vi "initialisationHWError.vi"(8 "error in (no error)":errorcluster, 11 "AtomChipHWC in":refnum<class "AtomChipHWC.lvclass">) -> (0 "error out":errorcluster, 3 "AtomChipHWC out":refnum<class "AtomChipHWC.lvclass">)   [LabVIEW 2011, in "Hardware.lvlib" / "HWControllers.lvlib" / "AtomChipHWC.lvclass"]
uses:
  AtomChipHWC.lvclass
  AtomChipHWC.lvclass/AtomChipHWC.ctl
  Channels/Digital/DigitalOutput.lvclass
  Channels/VoltOutput/AnalogOutput.lvclass
  Channels/DDSOutput/Generic/DDSOutput.lvclass
  Network Controllers/NetworkCamera/NetworkCamera.lvclass
  HWController.lvclass
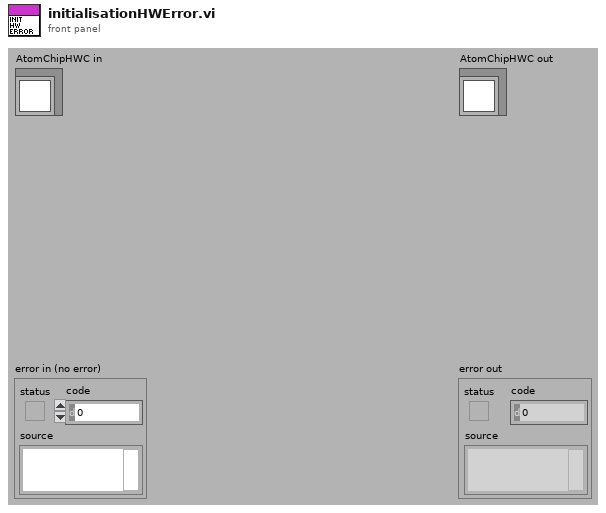
[diagram p1: front panel]
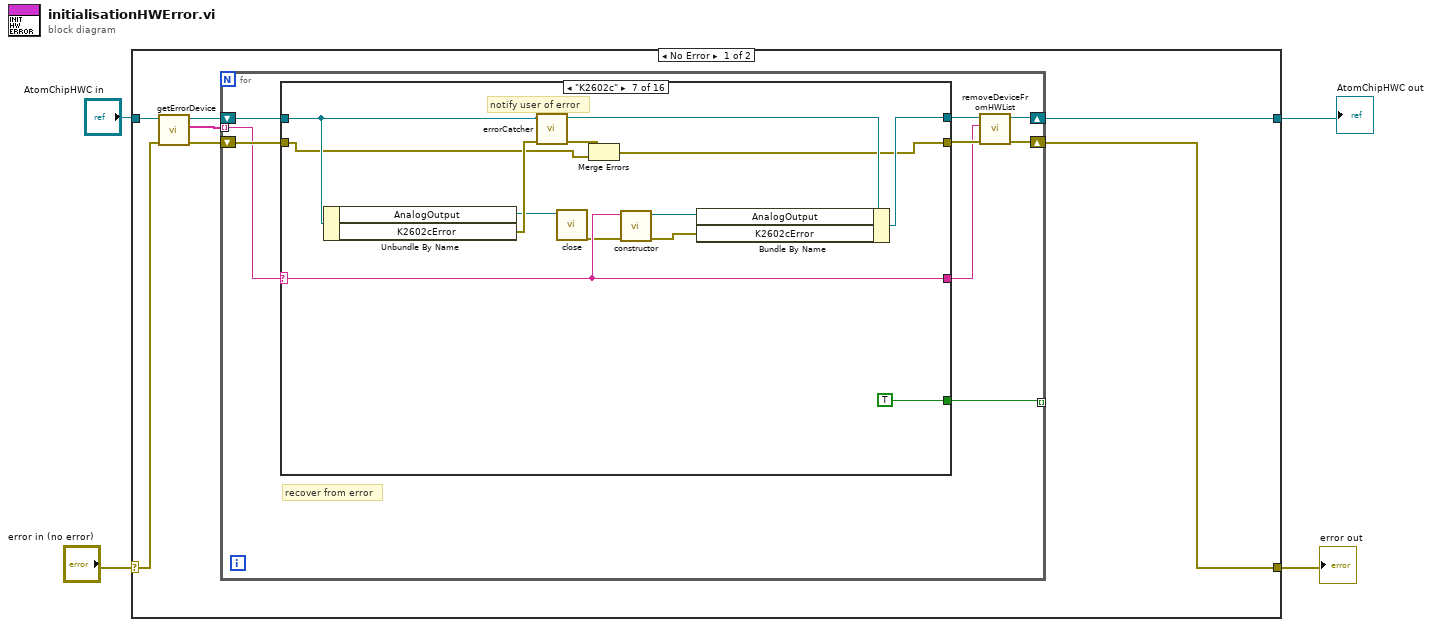
[diagram p0: block diagram]
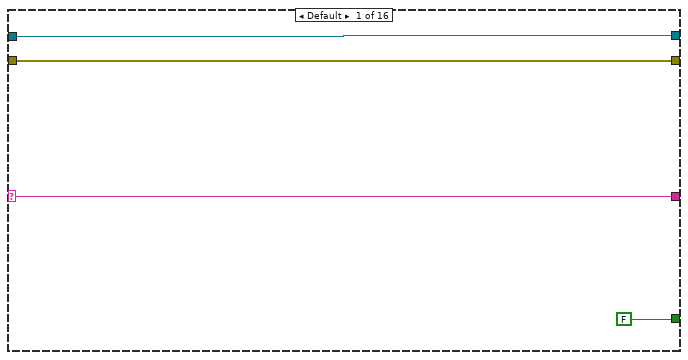
[diagram p2: hidden frame]
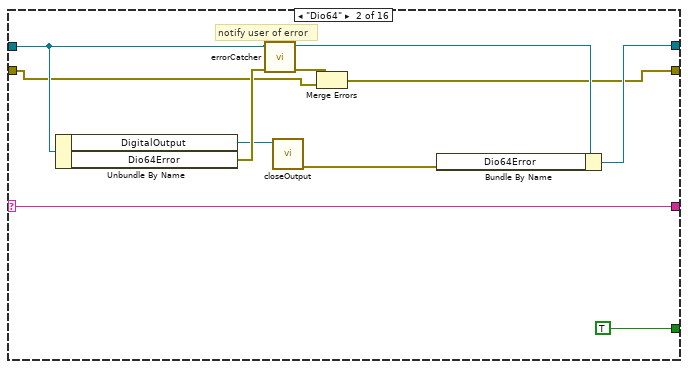
[diagram p3: hidden frame]
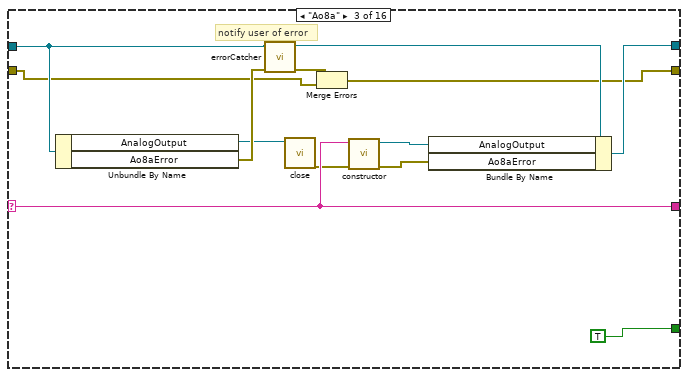
[diagram p4: hidden frame]
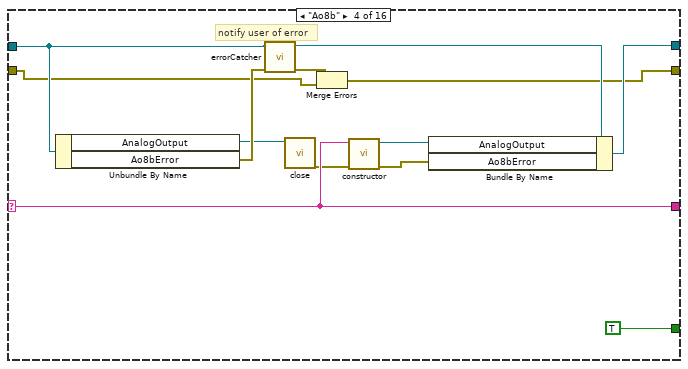
[diagram p5: hidden frame]
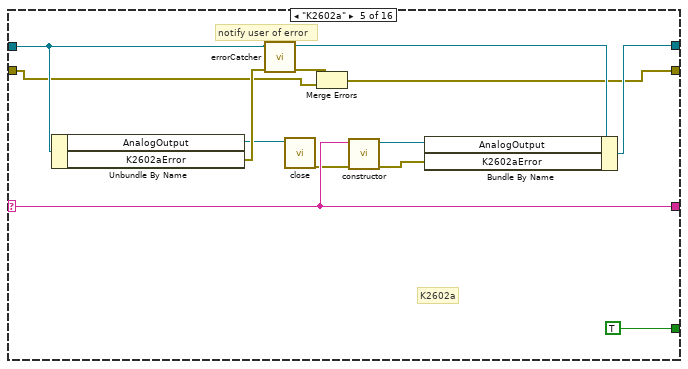
[diagram p6: hidden frame]
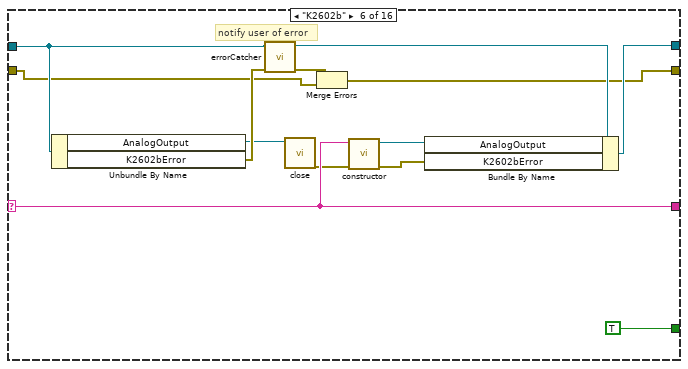
[diagram p7: hidden frame]
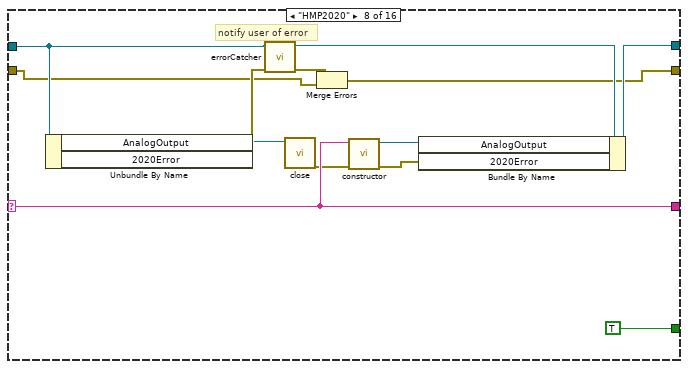
[diagram p8: hidden frame]
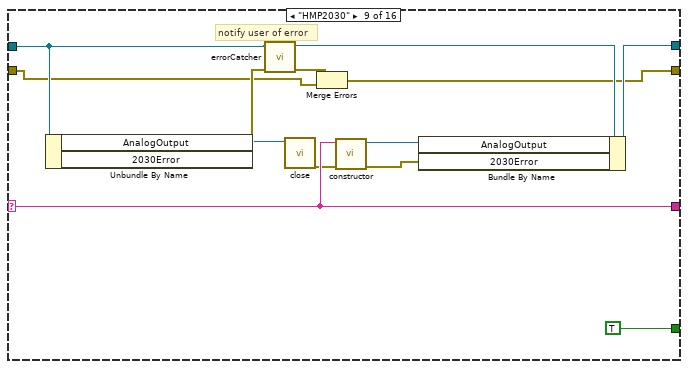
[diagram p9: hidden frame]
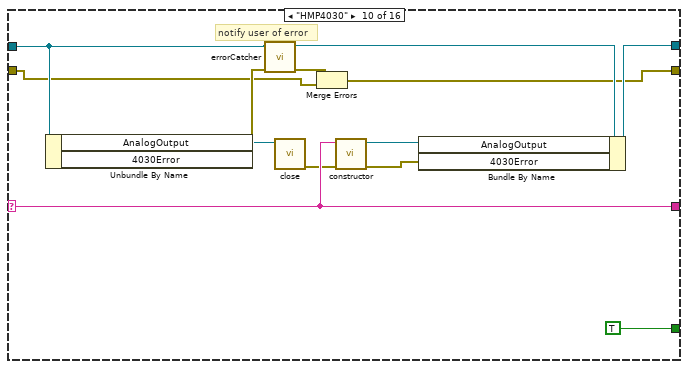
[diagram p10: hidden frame]
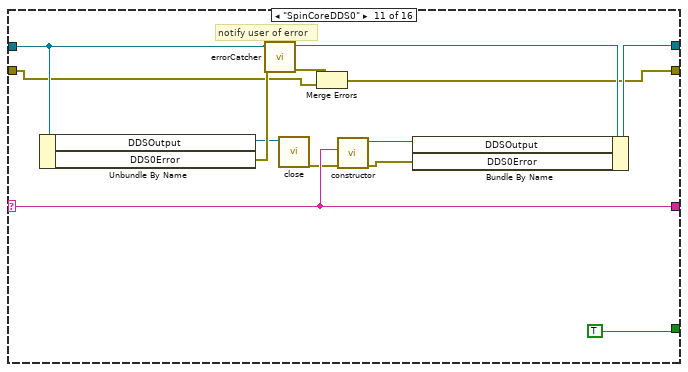
[diagram p11: hidden frame]
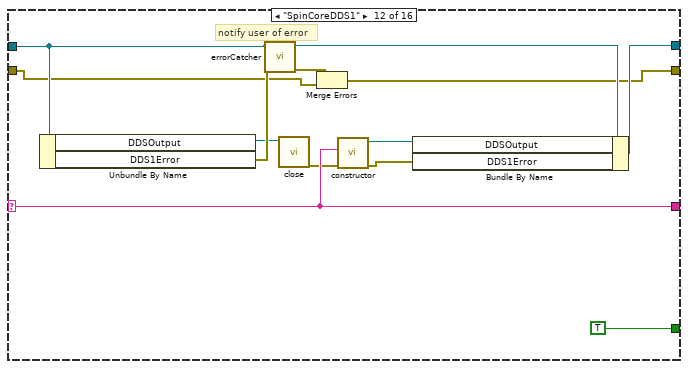
[diagram p12: hidden frame]
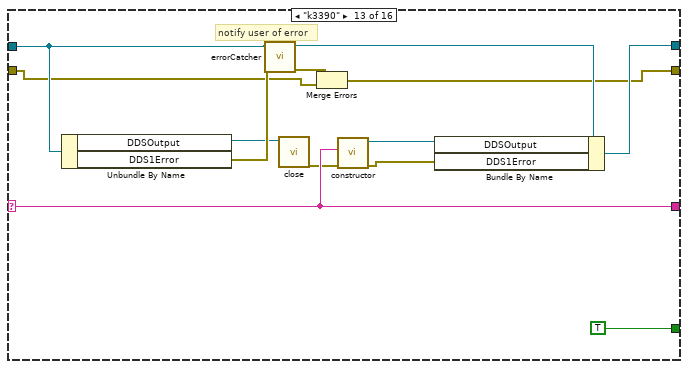
[diagram p13: hidden frame]
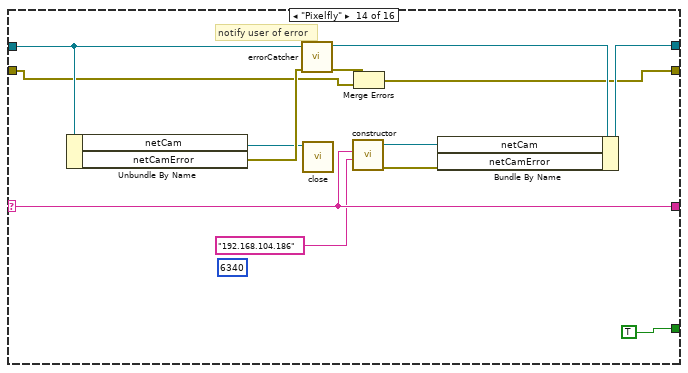
[diagram p14: hidden frame]
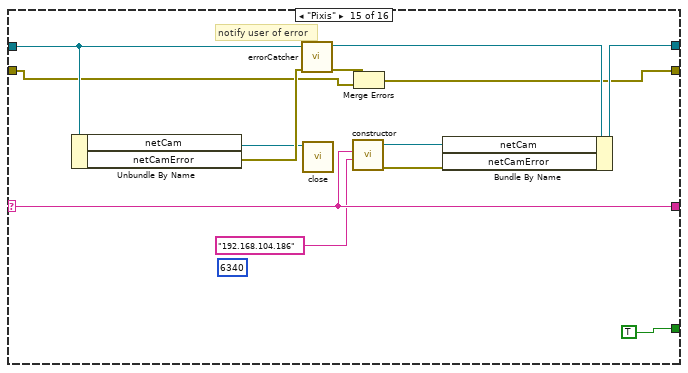
[diagram p15: hidden frame]
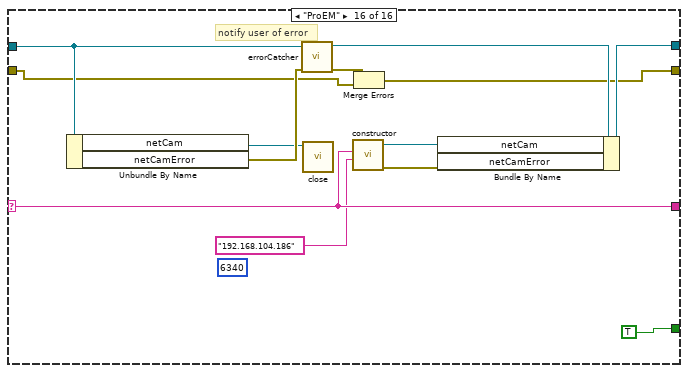
[diagram p16: hidden frame]
diagram:
  n1 = case shown="No Error" "error in (no error)" {
    selector: "error in (no error)" -> [w10 w218]
    tunnel: "AtomChipHWC in" -> [w11 w219]
    tunnel: [w6 w219] -> w2
    tunnel: [w5 w218] -> w1
    frame No Error {
      n2 = call "getErrorDevice.vi"("error in (no error)"=w10, "AtomChipHWC in"=w11) -> ("error out"=w7:errorcluster, "Devices"=w8:string[], "AtomChipHWC out"=w9:refnum<class "AtomChipHWC.lvclass">)  [unwired: 7 in]
      n3 = for {
        tunnel: w8 -> [w18] mode=indexing
        shift-right: [w14] -> w6
        shift-left: w9 -> [w20]
        shift-right: [w13] -> w5
        shift-left: w7 -> [w19]
        tunnel: [w12] -> _ mode=indexing
        # "recover from error"
        n4 = case shown="\"K2602c\"" w18 {
          selector: w18 -> [w22 w28 w40 w53 w66 w79 w92 w105 w118 w131 w142 w155 w168 w182 w195 w208]
          tunnel: w20 -> [w24 w35 w48 w61 w74 w87 w100 w113 w126 w139 w152 w165 w178 w191 w204 w217]
          tunnel: [w24 w30 w43 w56 w69 w82 w95 w108 w121 w134 w147 w160 w173 w186 w199 w212] -> w17
          tunnel: [w23 w29 w42 w55 w68 w81 w94 w107 w120 w133 w146 w159 w172 w185 w198 w211] -> w16
          tunnel: w19 -> [w23 w31 w44 w57 w70 w83 w96 w109 w122 w135 w148 w161 w174 w187 w200 w213]
          tunnel: [w22 w28 w40 w53 w66 w79 w92 w105 w118 w131 w142 w155 w168 w182 w195 w208] -> w15
          tunnel: [FALSE TRUE TRUE TRUE TRUE TRUE TRUE TRUE TRUE TRUE TRUE TRUE TRUE TRUE TRUE TRUE] -> w12
          frame Default {
          }
          frame "Dio64" {
            # "notify user of error"
            n5 = Unbundle By Name(w35) -> ("DigitalOutput"=w26:refnum<class "DigitalOutput.lvclass">, "Dio64Error"=w33:errorcluster)
            n6 = call-dynamic "errorCatcher.vi"("error in (no error)"=w33, "HWController in"=w35) -> ("error out"=w32:errorcluster, "HWController out"=w34:refnum<class "AtomChipHWC.lvclass">)  [unwired: 8 in]
            n7 = call-dynamic "closeOutput.vi"("DigitalOutput in"=w26) -> ("error out"=w27:errorcluster)  [unwired: 10 in]
            n8 = Merge Errors(w32, w31) -> (w29:errorcluster)
            n9 = Bundle By Name(cluster=w34, "Dio64Error"=w27) -> (w30:refnum<class "AtomChipHWC.lvclass">)
          }
          frame "Ao8a" {
            # "notify user of error"
            n10 = Unbundle By Name(w48) -> ("AnalogOutput"=w41:refnum<class "AnalogOutput.lvclass">, "Ao8aError"=w46:errorcluster)
            n11 = call-dynamic "errorCatcher.vi"("error in (no error)"=w46, "HWController in"=w48) -> ("error out"=w45:errorcluster, "HWController out"=w47:refnum<class "AtomChipHWC.lvclass">)  [unwired: 8 in]
            n12 = call-dynamic "close.vi"("AnalogOutput in"=w41) -> ("error out"=w39:errorcluster)  [unwired: 10 in]
            n13 = Merge Errors(w45, w44) -> (w42:errorcluster)
            n14 = call "constructor.vi"("error in (no error)"=w39, "deviceName"=w40) -> ("error out"=w37:errorcluster, "AnalogOutput out"=w38:refnum<class "AnalogOutput.lvclass">)  [unwired: 8 in]
            n15 = Bundle By Name(cluster=w47, "AnalogOutput"=w38, "Ao8aError"=w37) -> (w43:refnum<class "AtomChipHWC.lvclass">)
          }
          frame "Ao8b" {
            # "notify user of error"
            n16 = Unbundle By Name(w61) -> ("AnalogOutput"=w54:refnum<class "AnalogOutput.lvclass">, "Ao8bError"=w59:errorcluster)
            n17 = call-dynamic "errorCatcher.vi"("error in (no error)"=w59, "HWController in"=w61) -> ("error out"=w58:errorcluster, "HWController out"=w60:refnum<class "AtomChipHWC.lvclass">)  [unwired: 8 in]
            n18 = call-dynamic "close.vi"("AnalogOutput in"=w54) -> ("error out"=w52:errorcluster)  [unwired: 10 in]
            n19 = Merge Errors(w58, w57) -> (w55:errorcluster)
            n20 = call "constructor.vi"("error in (no error)"=w52, "deviceName"=w53) -> ("error out"=w50:errorcluster, "AnalogOutput out"=w51:refnum<class "AnalogOutput.lvclass">)  [unwired: 8 in]
            n21 = Bundle By Name(cluster=w60, "AnalogOutput"=w51, "Ao8bError"=w50) -> (w56:refnum<class "AtomChipHWC.lvclass">)
          }
          frame "K2602a" {
            # "K2602a"
            # "notify user of error"
            n22 = Unbundle By Name(w74) -> ("AnalogOutput"=w67:refnum<class "AnalogOutput.lvclass">, "K2602aError"=w72:errorcluster)
            n23 = call-dynamic "errorCatcher.vi"("error in (no error)"=w72, "HWController in"=w74) -> ("error out"=w71:errorcluster, "HWController out"=w73:refnum<class "AtomChipHWC.lvclass">)  [unwired: 8 in]
            n24 = call-dynamic "close.vi"("AnalogOutput in"=w67) -> ("error out"=w65:errorcluster)  [unwired: 10 in]
            n25 = Merge Errors(w71, w70) -> (w68:errorcluster)
            n26 = call "constructor.vi"("error in (no error)"=w65, "deviceName"=w66) -> ("error out"=w63:errorcluster, "AnalogOutput out"=w64:refnum<class "AnalogOutput.lvclass">)  [unwired: 8 in]
            n27 = Bundle By Name(cluster=w73, "AnalogOutput"=w64, "K2602aError"=w63) -> (w69:refnum<class "AtomChipHWC.lvclass">)
          }
          frame "K2602b" {
            # "notify user of error"
            n28 = Unbundle By Name(w87) -> ("AnalogOutput"=w80:refnum<class "AnalogOutput.lvclass">, "K2602bError"=w85:errorcluster)
            n29 = call-dynamic "errorCatcher.vi"("error in (no error)"=w85, "HWController in"=w87) -> ("error out"=w84:errorcluster, "HWController out"=w86:refnum<class "AtomChipHWC.lvclass">)  [unwired: 8 in]
            n30 = call-dynamic "close.vi"("AnalogOutput in"=w80) -> ("error out"=w78:errorcluster)  [unwired: 10 in]
            n31 = Merge Errors(w84, w83) -> (w81:errorcluster)
            n32 = call "constructor.vi"("error in (no error)"=w78, "deviceName"=w79) -> ("error out"=w76:errorcluster, "AnalogOutput out"=w77:refnum<class "AnalogOutput.lvclass">)  [unwired: 8 in]
            n33 = Bundle By Name(cluster=w86, "AnalogOutput"=w77, "K2602bError"=w76) -> (w82:refnum<class "AtomChipHWC.lvclass">)
          }
          frame "K2602c" {
            # "notify user of error"
            n34 = Unbundle By Name(w100) -> ("AnalogOutput"=w93:refnum<class "AnalogOutput.lvclass">, "K2602cError"=w98:errorcluster)
            n35 = call-dynamic "errorCatcher.vi"("error in (no error)"=w98, "HWController in"=w100) -> ("error out"=w97:errorcluster, "HWController out"=w99:refnum<class "AtomChipHWC.lvclass">)  [unwired: 8 in]
            n36 = call-dynamic "close.vi"("AnalogOutput in"=w93) -> ("error out"=w91:errorcluster)  [unwired: 10 in]
            n37 = Merge Errors(w97, w96) -> (w94:errorcluster)
            n38 = call "constructor.vi"("error in (no error)"=w91, "deviceName"=w92) -> ("error out"=w89:errorcluster, "AnalogOutput out"=w90:refnum<class "AnalogOutput.lvclass">)  [unwired: 8 in]
            n39 = Bundle By Name(cluster=w99, "AnalogOutput"=w90, "K2602cError"=w89) -> (w95:refnum<class "AtomChipHWC.lvclass">)
          }
          frame "HMP2020" {
            # "notify user of error"
            n40 = Unbundle By Name(w113) -> ("AnalogOutput"=w106:refnum<class "AnalogOutput.lvclass">, "2020Error"=w111:errorcluster)
            n41 = call-dynamic "errorCatcher.vi"("error in (no error)"=w111, "HWController in"=w113) -> ("error out"=w110:errorcluster, "HWController out"=w112:refnum<class "AtomChipHWC.lvclass">)  [unwired: 8 in]
            n42 = call-dynamic "close.vi"("AnalogOutput in"=w106) -> ("error out"=w104:errorcluster)  [unwired: 10 in]
            n43 = Merge Errors(w110, w109) -> (w107:errorcluster)
            n44 = call "constructor.vi"("error in (no error)"=w104, "deviceName"=w105) -> ("error out"=w102:errorcluster, "AnalogOutput out"=w103:refnum<class "AnalogOutput.lvclass">)  [unwired: 8 in]
            n45 = Bundle By Name(cluster=w112, "AnalogOutput"=w103, "2020Error"=w102) -> (w108:refnum<class "AtomChipHWC.lvclass">)
          }
          frame "HMP2030" {
            # "notify user of error"
            n46 = Unbundle By Name(w126) -> ("AnalogOutput"=w119:refnum<class "AnalogOutput.lvclass">, "2030Error"=w124:errorcluster)
            n47 = call-dynamic "errorCatcher.vi"("error in (no error)"=w124, "HWController in"=w126) -> ("error out"=w123:errorcluster, "HWController out"=w125:refnum<class "AtomChipHWC.lvclass">)  [unwired: 8 in]
            n48 = call-dynamic "close.vi"("AnalogOutput in"=w119) -> ("error out"=w117:errorcluster)  [unwired: 10 in]
            n49 = Merge Errors(w123, w122) -> (w120:errorcluster)
            n50 = call "constructor.vi"("error in (no error)"=w117, "deviceName"=w118) -> ("error out"=w115:errorcluster, "AnalogOutput out"=w116:refnum<class "AnalogOutput.lvclass">)  [unwired: 8 in]
            n51 = Bundle By Name(cluster=w125, "AnalogOutput"=w116, "2030Error"=w115) -> (w121:refnum<class "AtomChipHWC.lvclass">)
          }
          frame "HMP4030" {
            # "notify user of error"
            n52 = Unbundle By Name(w139) -> ("AnalogOutput"=w132:refnum<class "AnalogOutput.lvclass">, "4030Error"=w137:errorcluster)
            n53 = call-dynamic "errorCatcher.vi"("error in (no error)"=w137, "HWController in"=w139) -> ("error out"=w136:errorcluster, "HWController out"=w138:refnum<class "AtomChipHWC.lvclass">)  [unwired: 8 in]
            n54 = call-dynamic "close.vi"("AnalogOutput in"=w132) -> ("error out"=w130:errorcluster)  [unwired: 10 in]
            n55 = Merge Errors(w136, w135) -> (w133:errorcluster)
            n56 = call "constructor.vi"("error in (no error)"=w130, "deviceName"=w131) -> ("error out"=w128:errorcluster, "AnalogOutput out"=w129:refnum<class "AnalogOutput.lvclass">)  [unwired: 8 in]
            n57 = Bundle By Name(cluster=w138, "AnalogOutput"=w129, "4030Error"=w128) -> (w134:refnum<class "AtomChipHWC.lvclass">)
          }
          frame "SpinCoreDDS0" {
            # "notify user of error"
            n58 = Unbundle By Name(w152) -> ("DDSOutput"=w145:refnum<class "DDSOutput.lvclass">, "DDS0Error"=w150:errorcluster)
            n59 = call-dynamic "errorCatcher.vi"("error in (no error)"=w150, "HWController in"=w152) -> ("error out"=w149:errorcluster, "HWController out"=w151:refnum<class "AtomChipHWC.lvclass">)  [unwired: 8 in]
            n60 = call-dynamic "close.vi"("DDSOutput in"=w145) -> ("error out"=w141:errorcluster)  [unwired: 10 in]
            n61 = Merge Errors(w149, w148) -> (w146:errorcluster)
            n62 = call "constructor.vi"("error in (no error)"=w141, "device"=w142) -> ("error out"=w143:errorcluster, "DDSOutput out"=w144:refnum<class "DDSOutput.lvclass">)  [unwired: 8 in]
            n63 = Bundle By Name(cluster=w151, "DDSOutput"=w144, "DDS0Error"=w143) -> (w147:refnum<class "AtomChipHWC.lvclass">)
          }
          frame "SpinCoreDDS1" {
            # "notify user of error"
            n64 = Unbundle By Name(w165) -> ("DDSOutput"=w158:refnum<class "DDSOutput.lvclass">, "DDS1Error"=w163:errorcluster)
            n65 = call-dynamic "errorCatcher.vi"("error in (no error)"=w163, "HWController in"=w165) -> ("error out"=w162:errorcluster, "HWController out"=w164:refnum<class "AtomChipHWC.lvclass">)  [unwired: 8 in]
            n66 = call-dynamic "close.vi"("DDSOutput in"=w158) -> ("error out"=w154:errorcluster)  [unwired: 10 in]
            n67 = Merge Errors(w162, w161) -> (w159:errorcluster)
            n68 = call "constructor.vi"("error in (no error)"=w154, "device"=w155) -> ("error out"=w156:errorcluster, "DDSOutput out"=w157:refnum<class "DDSOutput.lvclass">)  [unwired: 8 in]
            n69 = Bundle By Name(cluster=w164, "DDSOutput"=w157, "DDS1Error"=w156) -> (w160:refnum<class "AtomChipHWC.lvclass">)
          }
          frame "k3390" {
            # "notify user of error"
            n70 = Unbundle By Name(w178) -> ("DDSOutput"=w171:refnum<class "DDSOutput.lvclass">, "DDS1Error"=w176:errorcluster)
            n71 = call-dynamic "errorCatcher.vi"("error in (no error)"=w176, "HWController in"=w178) -> ("error out"=w175:errorcluster, "HWController out"=w177:refnum<class "AtomChipHWC.lvclass">)  [unwired: 8 in]
            n72 = call-dynamic "close.vi"("DDSOutput in"=w171) -> ("error out"=w167:errorcluster)  [unwired: 10 in]
            n73 = Merge Errors(w175, w174) -> (w172:errorcluster)
            n74 = call "constructor.vi"("error in (no error)"=w167, "device"=w168) -> ("error out"=w169:errorcluster, "DDSOutput out"=w170:refnum<class "DDSOutput.lvclass">)  [unwired: 8 in]
            n75 = Bundle By Name(cluster=w177, "DDSOutput"=w170, "DDS1Error"=w169) -> (w173:refnum<class "AtomChipHWC.lvclass">)
          }
          frame "Pixelfly" {
            (unwired) u16 6340 ("remote port")
            # "notify user of error"
            n76 = Unbundle By Name(w191) -> ("netCam"=w179:refnum<class "NetworkCamera.lvclass">, "netCamError"=w189:errorcluster)
            n77 = call-dynamic "errorCatcher.vi"("error in (no error)"=w189, "HWController in"=w191) -> ("error out"=w188:errorcluster, "HWController out"=w190:refnum<class "AtomChipHWC.lvclass">)  [unwired: 8 in]
            n78 = call-dynamic "close.vi"("NetworkCamera in"=w179) -> ()  [unwired: 10 in, 1 out]
            n79 = call "constructor.vi"("machine name"="192.168.104.186" ("remote address"), "Camera"=w182) -> ("error out"=w180:errorcluster, "NetworkCamera out"=w183:refnum<class "NetworkCamera.lvclass">)  [unwired: 8 in]
            n80 = Merge Errors(w188, w187) -> (w185:errorcluster)
            n81 = Bundle By Name(cluster=w190, "netCam"=w183, "netCamError"=w180) -> (w186:refnum<class "AtomChipHWC.lvclass">)
          }
          frame "Pixis" {
            (unwired) u16 6340 ("remote port")
            # "notify user of error"
            n82 = Unbundle By Name(w204) -> ("netCam"=w192:refnum<class "NetworkCamera.lvclass">, "netCamError"=w202:errorcluster)
            n83 = call-dynamic "errorCatcher.vi"("error in (no error)"=w202, "HWController in"=w204) -> ("error out"=w201:errorcluster, "HWController out"=w203:refnum<class "AtomChipHWC.lvclass">)  [unwired: 8 in]
            n84 = call-dynamic "close.vi"("NetworkCamera in"=w192) -> ()  [unwired: 10 in, 1 out]
            n85 = call "constructor.vi"("machine name"="192.168.104.186" ("remote address"), "Camera"=w195) -> ("error out"=w193:errorcluster, "NetworkCamera out"=w196:refnum<class "NetworkCamera.lvclass">)  [unwired: 8 in]
            n86 = Merge Errors(w201, w200) -> (w198:errorcluster)
            n87 = Bundle By Name(cluster=w203, "netCam"=w196, "netCamError"=w193) -> (w199:refnum<class "AtomChipHWC.lvclass">)
          }
          frame "ProEM" {
            (unwired) u16 6340 ("remote port")
            # "notify user of error"
            n88 = Unbundle By Name(w217) -> ("netCam"=w205:refnum<class "NetworkCamera.lvclass">, "netCamError"=w215:errorcluster)
            n89 = call-dynamic "errorCatcher.vi"("error in (no error)"=w215, "HWController in"=w217) -> ("error out"=w214:errorcluster, "HWController out"=w216:refnum<class "AtomChipHWC.lvclass">)  [unwired: 8 in]
            n90 = call-dynamic "close.vi"("NetworkCamera in"=w205) -> ()  [unwired: 10 in, 1 out]
            n91 = call "constructor.vi"("machine name"="192.168.104.186" ("remote address"), "Camera"=w208) -> ("error out"=w206:errorcluster, "NetworkCamera out"=w209:refnum<class "NetworkCamera.lvclass">)  [unwired: 8 in]
            n92 = Merge Errors(w214, w213) -> (w211:errorcluster)
            n93 = Bundle By Name(cluster=w216, "netCam"=w209, "netCamError"=w206) -> (w212:refnum<class "AtomChipHWC.lvclass">)
          }
        }
        n94 = call "removeDeviceFromHWList.vi"("error in (no error)"=w16, "deviceName"=w15, "HWController in"=w17) -> ("error out"=w13:errorcluster, "HWController out"=w14:refnum<class "AtomChipHWC.lvclass">)  [unwired: 7 in]
      }
    }
    frame Error {
    }
  }
  "error out" <- w1
  "AtomChipHWC out" <- w2
